vi "SaveData.vi"(0 "CSV Logging in":refnum<class "CSV Logging.lvclass">, 1 "Path Control":path, 2 "Signal":dbl[](graph), 3 "error in (no error)":errorcluster) -> (7 "CSV Logging out":refnum<class "CSV Logging.lvclass">, 10 "error out":errorcluster)   [LabVIEW 2020, in "CSV Logging.lvlib" / "CSV Logging.lvclass"]
uses:
  CSV Logging.lvclass
  <vilib>/Utility/file.llb/Write Delimited Spreadsheet (DBL).vi
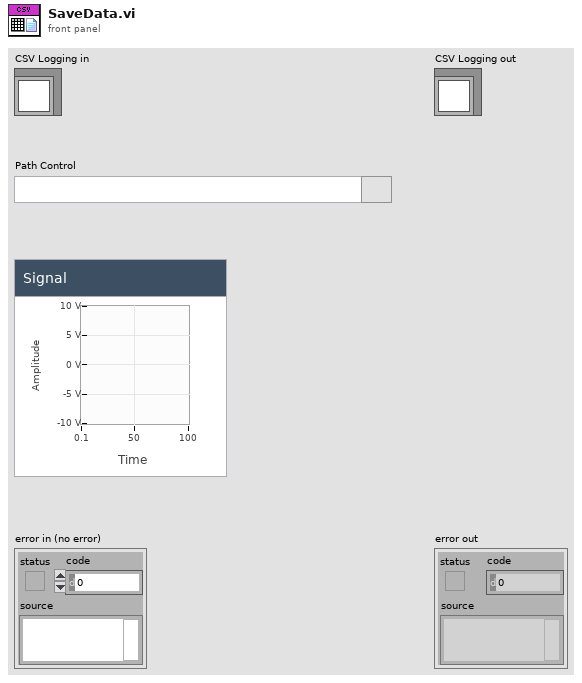
[diagram p1: front panel]
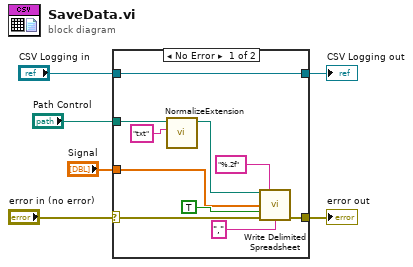
[diagram p0: block diagram]
diagram:
  n1 = case shown="No Error" "error in (no error)" {
    selector: "error in (no error)" -> [w11 w17]
    tunnel: "CSV Logging in" -> [w16 w18]
    tunnel: [w16 w18] -> w5
    tunnel: [w12 w17] -> w3
    tunnel: "Path Control" -> [w15 _]
    tunnel: "Signal" -> [w7 _]
    frame No Error {
      n2 = call "NormalizeExtension.vi"("Extension"="txt", "Path in"=w15) -> ("Path out"=w13:path)  [unwired: 9 in]
      n3 = call-poly <vilib>:"Write Delimited Spreadsheet.vi"("file path (dialog if empty)"=w13, "format (%.3f)"="%.2f", "1D data"=w7, "append to file? (new file:F)"=TRUE, "error in (no error)"=w11, "delimiter (\\t)"="," ("delimiter (\\t)")) -> ("error out"=w12:errorcluster)  [unwired: 8 in, 1 out]
    }
    frame Error {
    }
  }
  "error out" <- w3
  "CSV Logging out" <- w5
